vi "PH_AWG-510.Store wanted Output Settings.vi"(0 "VI in":refnum<vi>, 2 "Wanted Output Settings":T1={"Activate Channel"=FALSE, "VPP (V)"=0.0, "Clock (Hz)"=0.0, "File Name (Device)"="", "#1"=0, "#2"=0, "#3"=0, "#4"=0, "#5"=0, "#6"=0, "#7"=0, "#8"=0, "#9"=0, "#10"=0, "#11"=0, "#12"=0, "#13"=0, "#14"=0, "#15"=0, "#16"=0, "#17"=0, "#18"=0, "#19"=0, "#20"=0, "Offset (V)"=-1.0} {"#20" max=1023 step=1 scale=0.0..1023.0; "#19" max=1023 step=1 scale=0.0..1023.0; "#18" max=1023 step=1 scale=0.0..1023.0; "#17" max=1023 step=1 scale=0.0..1023.0; "#16" max=1023 step=1 scale=0.0..1023.0; "#15" max=1023 step=1 scale=0.0..1023.0; "#14" max=1023 step=1 scale=0.0..1023.0; "#13" max=1023 step=1 scale=0.0..1023.0; "#12" max=1023 step=1 scale=0.0..1023.0; "#11" max=1023 step=1 scale=0.0..1023.0; "#10" max=1023 step=1 scale=0.0..1023.0; "#9" max=1023 step=1 scale=0.0..1023.0; "#8" max=1023 step=1 scale=0.0..1023.0; "#7" max=1023 step=1 scale=0.0..1023.0; "#6" max=1023 step=1 scale=0.0..1023.0; "#5" max=1023 step=1 scale=0.0..1023.0; "#4" max=1023 step=1 scale=0.0..1023.0; "#3" max=1023 step=1 scale=0.0..1023.0; "#2" max=1023 step=1 scale=0.0..1023.0; "#1" max=1023 step=1 scale=0.0..1023.0}, 5 "error in (no error)":errorcluster) -> (14 "VI out":refnum<vi>, 19 "error out":errorcluster)   [LabVIEW 2014, in "PH_AWG-510.lvlib"]
doc: "This VI writes wanted Output Settings to own attributes if they are different."
uses:
  PH_AWG-510.lvlib
  PH_AWG-510.Output Settings.ctl
panel:
  # "Waveform Pattern"
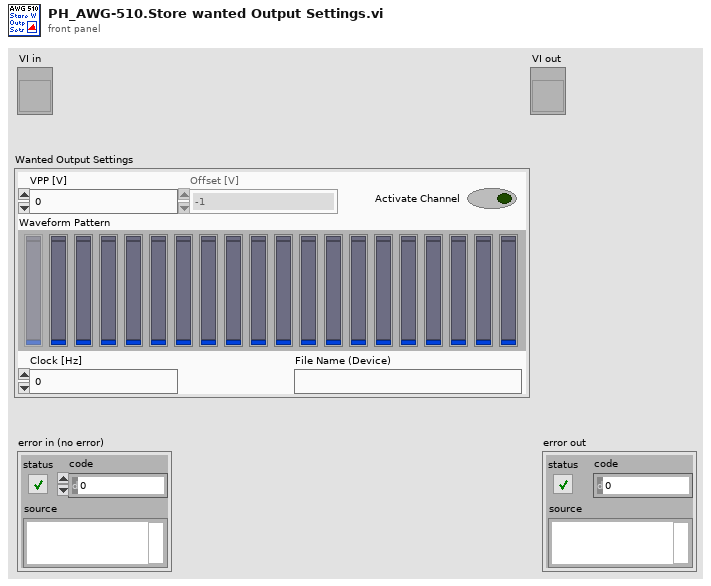
[diagram p1: front panel]
types:
  T1 = typedef "PH_AWG-510.lvlib/PH_AWG-510.Output Settings.ctl" = cluster{"Activate Channel":bool, "VPP (V)":dbl, "Clock (Hz)":dbl, "File Name (Device)":string, "#1":u16, "#2":u16, "#3":u16, "#4":u16, "#5":u16, "#6":u16, "#7":u16, "#8":u16, "#9":u16, "#10":u16, "#11":u16, "#12":u16, "#13":u16, "#14":u16, "#15":u16, "#16":u16, "#17":u16, "#18":u16, "#19":u16, "#20":u16, "Offset (V)":dbl}
  T2 = typedef "PH_AWG-510.lvlib/PH_AWG-510.i attribute.ctl" = cluster{"GUI Refs":cluster{"Delete":refnum<vi>, "Trigger Settings":refnum<vi>, "Start Device":refnum<vi>, "Instrument Information":refnum<vi>, "Lock Frontpanel":refnum<vi>, "Waveform Pattern File":refnum<vi>, "Initialize":refnum<vi>, "Output Settings":refnum<vi>}, "Instrument Information":T3, "Initialized?":bool, "Current Settings":cluster{"Trigger":T4, "Output Settings":T1}, "Wanted Settings":cluster{"Trigger":T4, "Output Settings":T1}, "Device frontpanel locked?":bool, "Default File Path":path}
  T3 = typedef "PH_AWG-510.lvlib/PH_AWG-510.Instrument Information Dataset.ctl" = cluster{"VISA resource name":refnum<visa-resource-name>, "Instrument Firmware Revision":string, "Manufacturer":string, "Model":string, "Serial Number":string, "Error Message":string, "Device Status":enum16{"stopped", "wating for trigger", "running", "Failure"}}
  T4 = typedef "PH_AWG-510.lvlib/PH_AWG-510.Trigger Settings.ctl" = cluster{"Mode":enum16{"Continuous", "Triggered", "Gated", "Enhanced"}, "Level (V)":dbl, "External Source":bool}
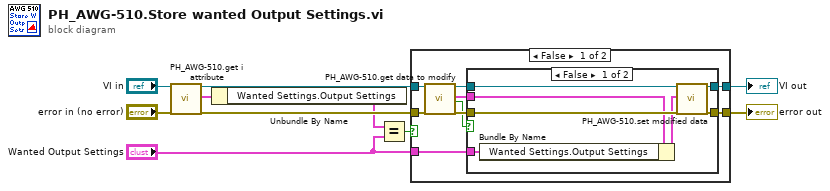
[diagram p0: block diagram]
diagram:
  n1 = call "PH_AWG-510.get i attribute.vi"("i ref in"="VI in", "error in (no error)"="error in (no error)") -> ("i ref out"=w7:refnum<vi>, "i attribute"=w3:T2, "error out"=w4:errorcluster)  [unwired: 15 in]
  n2 = Unbundle By Name(w3) -> ("Wanted Settings.Output Settings"=w2:T1)
  n3 = Equal?(x=w2, y="Wanted Output Settings") -> (x = y?=w10:bool)
  n4 = case shown="False" w10 {
    tunnel: w4 -> [w19 w29]
    tunnel: [w17 w29] -> w8
    tunnel: w7 -> [w16 w30]
    tunnel: "Wanted Output Settings" -> [w13 _]
    tunnel: [w11 w30] -> w9
    frame False {
      n5 = call "PH_AWG-510.get data to modify.vi"("i ref in"=w16, "error in (no error)"=w19) -> ("i ref out"=w15:refnum<vi>, "i attribute"=w14:T2, "timed out"=w12:bool, "error out"=w18:errorcluster)  [unwired: 14 in]
      n6 = case shown="False" w12 {
        tunnel: w18 -> [w26 w28]
        tunnel: [w25 w28] -> w17
        tunnel: w15 -> [w24 w27]
        tunnel: w14 -> [w23 _]
        tunnel: w13 -> [w20 _]
        tunnel: [w21 w27] -> w11
        frame False {
          n7 = Bundle By Name(cluster=w23, "Wanted Settings.Output Settings"=w20) -> (w22:T2)
          n8 = call "PH_AWG-510.set modified data.vi"("i ref in"=w24, "i attribute"=w22, "error in (no error)"=w26) -> ("i ref out"=w21:refnum<vi>, "error out"=w25:errorcluster)  [unwired: 15 in]
        }
        frame True {
        }
      }
    }
    frame True {
    }
  }
  "VI out" <- w9
  "error out" <- w8
